vi "Build State Change Action.vi"(4 "Current State":variant, 5 "Target State":variant) -> (1 "Action String Out":string)   [LabVIEW 2016]
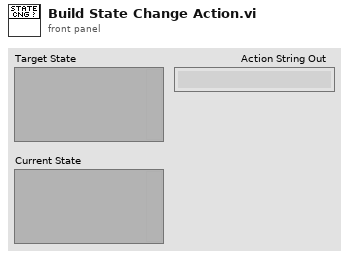
[diagram p1: front panel]
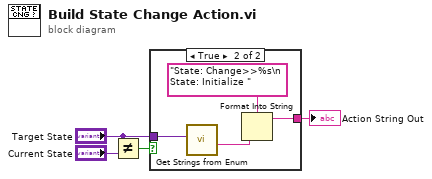
[diagram p0: block diagram]
diagram:
  n1 = Not Equal?(x="Target State", y="Current State") -> (x != y?=w1:bool)
  n2 = case shown="True" w1 {
    tunnel: [_ w6] -> w2
    tunnel: "Target State" -> [_ w8]
    frame False {
    }
    frame True {
      n3 = call "Get Strings from Enum.vi"("Enum"=w8) -> ("String Value"=w5:string)  [unwired: 7 in, 3 out]
      n4 = Format Into String(format string="State: Change>>%s\n State: Initialize " ("State(s) at Back (\"\")"), w5) -> (resulting string=w6:string)  [unwired: 2 in, 1 out]
    }
  }
  "Action String Out" <- w2
